vi "Parse TCP-IP Response 4_RED.vi"(0 "TCP/IP ID":refnum<k5>, 7 "timeout ms (5000)":i32=5000, 11 "error in (no error)":errorcluster) -> (1 "Header":string, 2 "Packet Error Code":i32, 3 "Packet ID":u8, 4 "Data Type":u16, 6 "Command Done":cluster{"Function #":u16}, 8 "Acq. Status":T3, 10 "Image Packet":T2, 12 "Status Array":string[](array[string]), 13 "Camera ID":u8, 14 "SI Image Settings":T1, 15 "error out":errorcluster)   [LabVIEW 2015]
uses:
  TCP-IP Image Packet.ctl
  SI Image Settings 1.ctl
panel:
  out "Data Bytes":i32
  out "String":string
  out "TCP/IP String":string
  out "Packet Length":u32
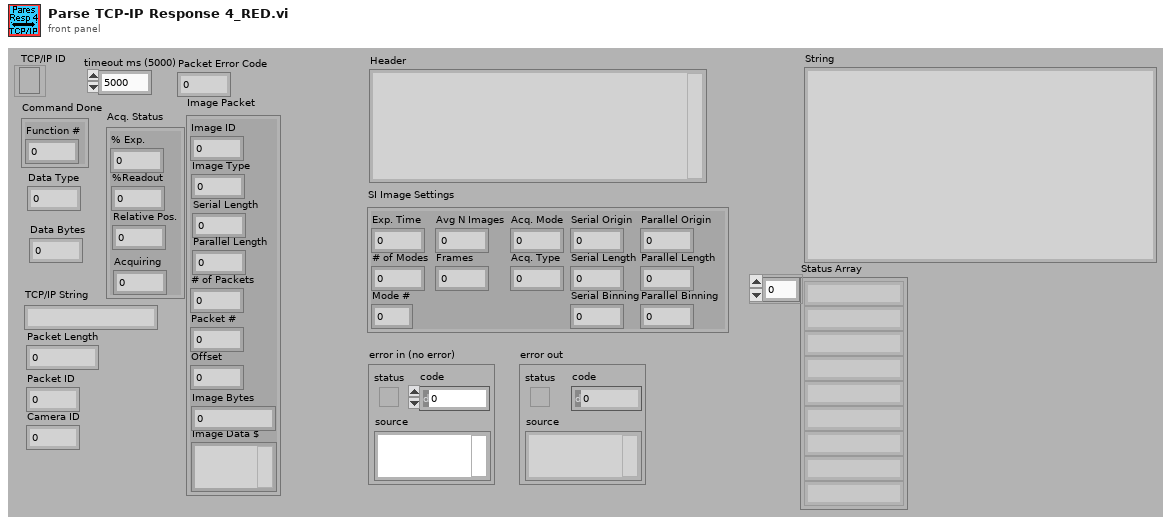
[diagram p1: front panel]
types:
  T1 = typedef "SI Image Settings 1.ctl" = cluster{"Exp. Time":u32, "# of Modes":u8, "Mode #":u8, "Avg N Images":u32, "Frames":u32, "Acq. Mode":u16, "Acq. Type":u16, "Serial Origin":i32, "Serial Length":i32, "Serial Binning":i32, "Parallel Origin":i32, "Parallel Length":i32, "Parallel Binning":i32}
  T2 = typedef "TCP-IP Image Packet.ctl" = cluster{"Image ID":u16, "Image Type":u16, "Serial Length":u16, "Parallel Length":u16, "# of Packets":u16, "Packet #":u16, "Offset":u32, "Image Bytes":u32, "Image Data $":string}
  T3 = cluster{"% Exp.":u16, "%Readout":u16, "Relative Pos.":u32, "Acquiring":i32}
  T4 = enum16{"Standard", "Buffered", "CRLF", "Immediate"}
  T5 = cluster{"Image ID":u16, "Image Type":u16, "Serial Length":u16, "Parallel Length":u16, "# of Packets":i32, "Packet #":i32, "Offset":i32, "Image Bytes":u32}
  T6 = cluster{"Image ID":u16, "Image Type":u16, "Serial Length":u16, "Parallel Length":u16, "# of Packets":i32, "Packet #":i32, "Offset":i32, "Image Bytes":u32, "data out":string}
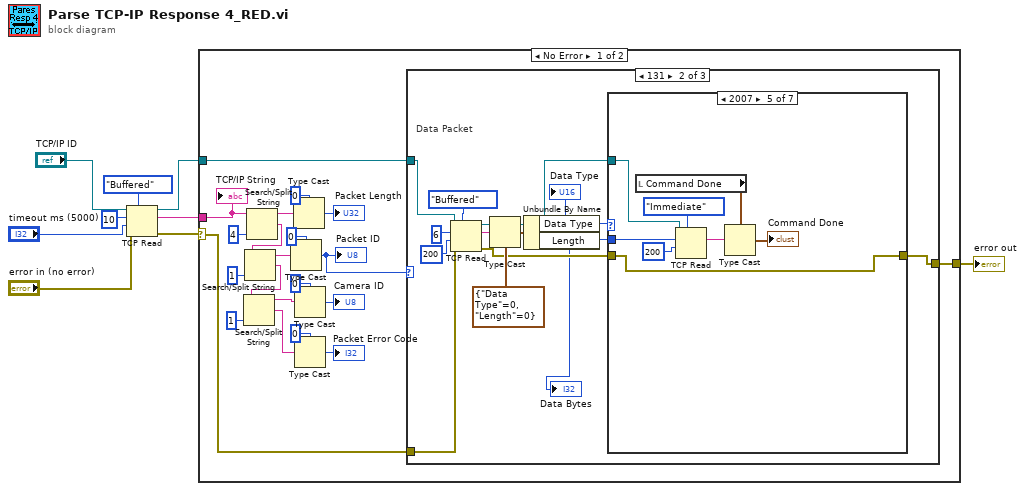
[diagram p0: block diagram]
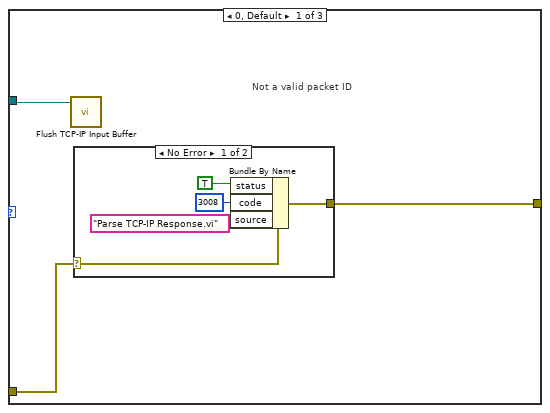
[diagram p2: hidden frame]
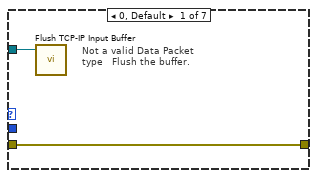
[diagram p4: hidden frame]
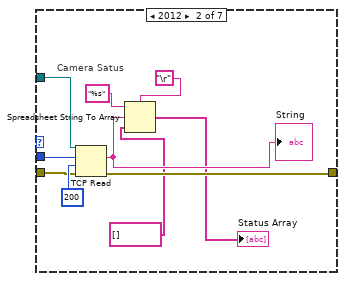
[diagram p5: hidden frame]
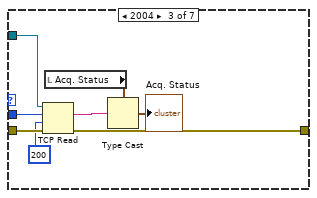
[diagram p6: hidden frame]
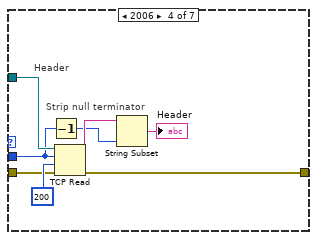
[diagram p7: hidden frame]
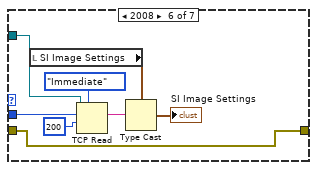
[diagram p8: hidden frame]
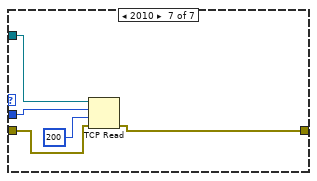
[diagram p9: hidden frame]
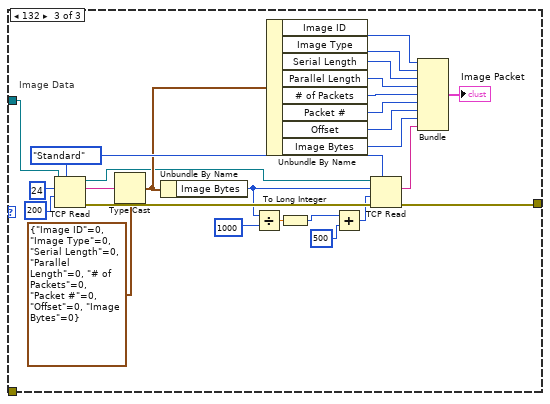
[diagram p10: hidden frame]
diagram:
  n1 = TCP Read(connection ID="TCP/IP ID", bytes to read=10, error in (no error)="error in (no error)", 7:T4."Buffered" ("mode (standard)"), 9:"timeout ms (5000)") -> (connection ID out=w1:refnum<k5>, data out=w7:string, error out=w3:errorcluster)
  n2 = case shown="No Error" w3 {
    selector: w3 -> [w16 w128]
    tunnel: w7 -> [w20 _]
    tunnel: w1 -> [w18 _]
    tunnel: [w17 w128] -> w5
    frame No Error {
      n3 = Search/Split String(string=w20, offset (0)=4) -> (substring before match=w24:string, match + rest of string=w23:string)  [unwired: 1 in, 1 out]
      n4 = Search/Split String(string=w23, offset (0)=u16 1 ("default (0L)")) -> (substring before match=w25:string, match + rest of string=w14:string)  [unwired: 1 in, 1 out]
      n5 = Search/Split String(string=w14, offset (0)=u16 1 ("default (0L)")) -> (substring before match=w13:string, match + rest of string=w11:string)  [unwired: 1 in, 1 out]
      n6 = Type Cast(type=u8 0 ("default (0L)"), x=w25) -> (*(type *) &x=w19:u8)
      "Packet ID" <- w19
      n7 = Type Cast(type=u32 0 ("default (0L)"), x=w24) -> (*(type *) &x=→"Packet Length":u32)
      n8 = Type Cast(type=u8 0 ("default (0L)"), x=w13) -> (*(type *) &x=→"Camera ID":u8)
      n9 = Type Cast(type=0 ("default (0L)"), x=w11) -> (*(type *) &x=→"Packet Error Code":i32)
      n10 = case shown="131" w19 {
        tunnel: w18 -> [w31 w44 w110]
        tunnel: w16 -> [w32 w49 _]
        tunnel: [w33 w42 w122] -> w17
        frame 0, Default {
          # "Not a valid packet ID"
          n11 = call "Flush TCP-IP Input Buffer.vi"("TCP/IP ID"=w31) -> ()  [unwired: 4 in, 1 out]
          n12 = case shown="No Error" w32 {
            selector: w32 -> [w34 w39]
            tunnel: [w38 w39] -> w33
            frame No Error {
              n13 = Bundle By Name(cluster=w34, "status"=TRUE, "code"=3008, "source"="Parse TCP-IP Response.vi") -> (w38:errorcluster)
            }
            frame Error {
            }
          }
        }
        frame 131 {
          # "Data Packet"
          n14 = TCP Read(connection ID=w44, bytes to read=6, error in (no error)=w49, 7:T4."Buffered" ("mode (standard)"), 9:200 ("timeout ms (25000)")) -> (connection ID out=w40:refnum<k5>, data out=w48:string, error out=w43:errorcluster)
          n15 = Type Cast(type=cluster{"Data Type":u16, "Length":i32} {"Data Type"=0, "Length"=0}, x=w48) -> (*(type *) &x=w46:cluster{"Data Type":u16, "Length":i32})
          n16 = Unbundle By Name(w46) -> ("Data Type"=w45:u16, "Length"=w41:i32)
          "Data Type" <- w45
          "Data Bytes" <- w41
          n17 = case shown="2007" w45 {
            tunnel: w40 -> [w53 w61 w72 w77 w83 w92 w99]
            tunnel: w41 -> [_ w62 w71 w75 w82 w91 w100]
            tunnel: w43 -> [w54 w63 w70 w79 w81 w90 w98]
            tunnel: [w54 w60 w68 w78 w81 w90 w97] -> w42
            frame 0, Default {
              # "Not a valid Data Packet type   Flush the buffer."
              n18 = call "Flush TCP-IP Input Buffer.vi"("TCP/IP ID"=w53) -> ()  [unwired: 4 in, 1 out]
            }
            frame 2012 {
              # "Camera Satus"
              n19 = TCP Read(connection ID=w61, bytes to read=w62, error in (no error)=w63, 9:200 ("timeout ms (25000)")) -> (data out=w58:string, error out=w60:errorcluster)  [unwired: 1 in, 1 out]
              "String" <- w58
              n20 = Spreadsheet String To Array(delimiter (Tab)="\r", format string="%s", spreadsheet string=w58, array type (2D Dbl)=string[] []) -> (array=→"Status Array":string[])
            }
            frame 2004 {
              n21 = TCP Read(connection ID=w72, bytes to read=w71, error in (no error)=w70, 9:200 ("timeout ms (25000)")) -> (data out=w69:string, error out=w68:errorcluster)  [unwired: 1 in, 1 out]
              n22 = local read "Acq. Status"() -> (w65:T3)
              n23 = Type Cast(type=w65, x=w69) -> (*(type *) &x=→"Acq. Status":T3)
            }
            frame 2006 {
              # "Strip null terminator"
              # "Header"
              n24 = Decrement(x=w75) -> (x-1=w74:i32)
              n25 = TCP Read(connection ID=w77, bytes to read=w75, error in (no error)=w79, 9:200 ("timeout ms (25000)")) -> (data out=w76:string, error out=w78:errorcluster)  [unwired: 1 in, 1 out]
              n26 = String Subset(string=w76, length (rest)=w74) -> (substring=→"Header":string)  [unwired: 1 in]
            }
            frame 2007 {
              n27 = local read "Command Done"() -> (w85:cluster{"Function #":u16})
              n28 = TCP Read(connection ID=w83, bytes to read=w82, 7:T4."Immediate" ("mode (standard)"), 9:200 ("timeout ms (25000)")) -> (data out=w86:string)  [unwired: 1 in, 2 out]
              n29 = Type Cast(type=w85, x=w86) -> (*(type *) &x=→"Command Done":cluster{"Function #":u16})
            }
            frame 2008 {
              n30 = local read "SI Image Settings"() -> (w93:T1)
              n31 = TCP Read(connection ID=w92, bytes to read=w91, 7:T4."Immediate" ("mode (standard)"), 9:200 ("timeout ms (25000)")) -> (data out=w94:string)  [unwired: 1 in, 2 out]
              n32 = Type Cast(type=w93, x=w94) -> (*(type *) &x=→"SI Image Settings":T1)
            }
            frame 2010 {
              n33 = TCP Read(connection ID=w99, bytes to read=w100, error in (no error)=w98, 9:200 ("timeout ms (25000)")) -> (error out=w97:errorcluster)  [unwired: 1 in, 2 out]
            }
          }
        }
        frame 132 {
          w126 = T4."Standard" ("mode (standard)")
          # "Image Data"
          n34 = TCP Read(connection ID=w110, bytes to read=24, 7:w126, 9:200 ("timeout ms (25000)")) -> (connection ID out=w111:refnum<k5>, data out=w124:string, error out=w123:errorcluster)  [unwired: 1 in]
          n35 = Type Cast(type=T5 {"Image ID"=0, "Image Type"=0, "Serial Length"=0, "Parallel Length"=0, "# of Packets"=0, "Packet #"=0, "Offset"=0, "Image Bytes"=0} ("*(type *) &x"), x=w124) -> (*(type *) &x=w112:T5)
          n36 = Unbundle By Name(w112) -> ("Image Bytes"=w109:u32)
          n37 = Divide(x=w109, y=1000 ("timeout ms (25000)")) -> (x/y=w107:dbl)
          n38 = Unbundle By Name(w112) -> ("Image ID"=w120:u16, "Image Type"=w119:u16, "Serial Length"=w118:u16, "Parallel Length"=w117:u16, "# of Packets"=w116:i32, "Packet #"=w115:i32, "Offset"=w105:i32, "Image Bytes"=w104:u32)
          n39 = To Long Integer(number=w107) -> (32bit integer=w106:i32)
          n40 = Add(x=w106, y=500) -> (x+y=w103:i32)
          n41 = TCP Read(connection ID=w111, bytes to read=w109, error in (no error)=w123, 7:w126, 9:w103) -> (data out=w114:string, error out=w122:errorcluster)  [unwired: 1 out]
          n42 = Bundle("Image ID"=w120, "Image Type"=w119, "Serial Length"=w118, "Parallel Length"=w117, "# of Packets"=w116, "Packet #"=w115, "Offset"=w105, "Image Bytes"=w104, "data out"=w114) -> (→"Image Packet":T6)  [unwired: 1 in]
        }
      }
      "TCP/IP String" <- w20
    }
    frame Error {
    }
  }
  "error out" <- w5
